vi "Robot参数整合一.vi"(7 "M4A数据":string[](array[string])=["", "", "", "", ""], 8 "A_Robot数据":string[](array[string])=["", "", "", "", "", "", "", "", "", "", "", "", "", "", ""], 10 "良率结算结果":string[](array[string]), 11 "Robot参数输入":string[](array[string])) -> (0 "Total数":string, 2 "数据整合输出":string[](array[string]), 3 "Robot数据输出结果":string[](array[string]))   [LabVIEW 2011]
panel:
  in  "数组":string[](array[string])=["Robot IP Set", "Robot Port Set", "PLC IP Set", "PLC Port Set", "Title Path", "Product", "StationID", "MachineSN", "HW", "GUI-Ver", "Robot-Ver", "Vision-Ver", "MachinMAC"]
  # "Product\n\nSN\n\nStationID\nMachineSN\nHW\nGUI-Ver\nRobot-Ver\nVision-Ver\n\nIP\n\nMachinMAC\n\nM4 Result\t\nblack wifi杓0.0\nM4 Fixture 1\n\nPoint,X,Y,Angle\nStartTime\nEndTime\nTime of CCD photographing\nM4 FPYR\nM4 Failing Rate\nM4 ReTest\nM4 CumRetestYield\nM4 ThroughtRate"
  # "Product\t\nStationID\t\nMachineSN\t\nHW\t\nGUI-Ver\t\nRobot-Ver\t\nVision-Ver\t\nIP\t\nMachinMAC\t\nPoint,X,Y,Angle\t\nStartTime\t\nEndTime\t\nTime of CCD photographing\t\nM4 FPYR\t\nM4 Failing Rate\t\nM4 ReTest\t\nM4 CumRetestYield\t\nM4 ThroughtRate\t\nRobot-OriginPosition\t\nRobot-CCD TopPosition\t\nRobot-CCD OriginPosition\t\nRobot-CCD ReTopPosition\t\nRobot-M4 TopPosition\t\nRobot-M4 OriginPosition\t\nRobot_M4 ReTopPosition\t\nRobot_CurrentPosition\t\nRobot-M4 TopPosition\t\nRobot-M4 OriginPosition\t\nRobot-M4 TopPosition\t\nM4_PassPosition\t\nM4_FailPosition"
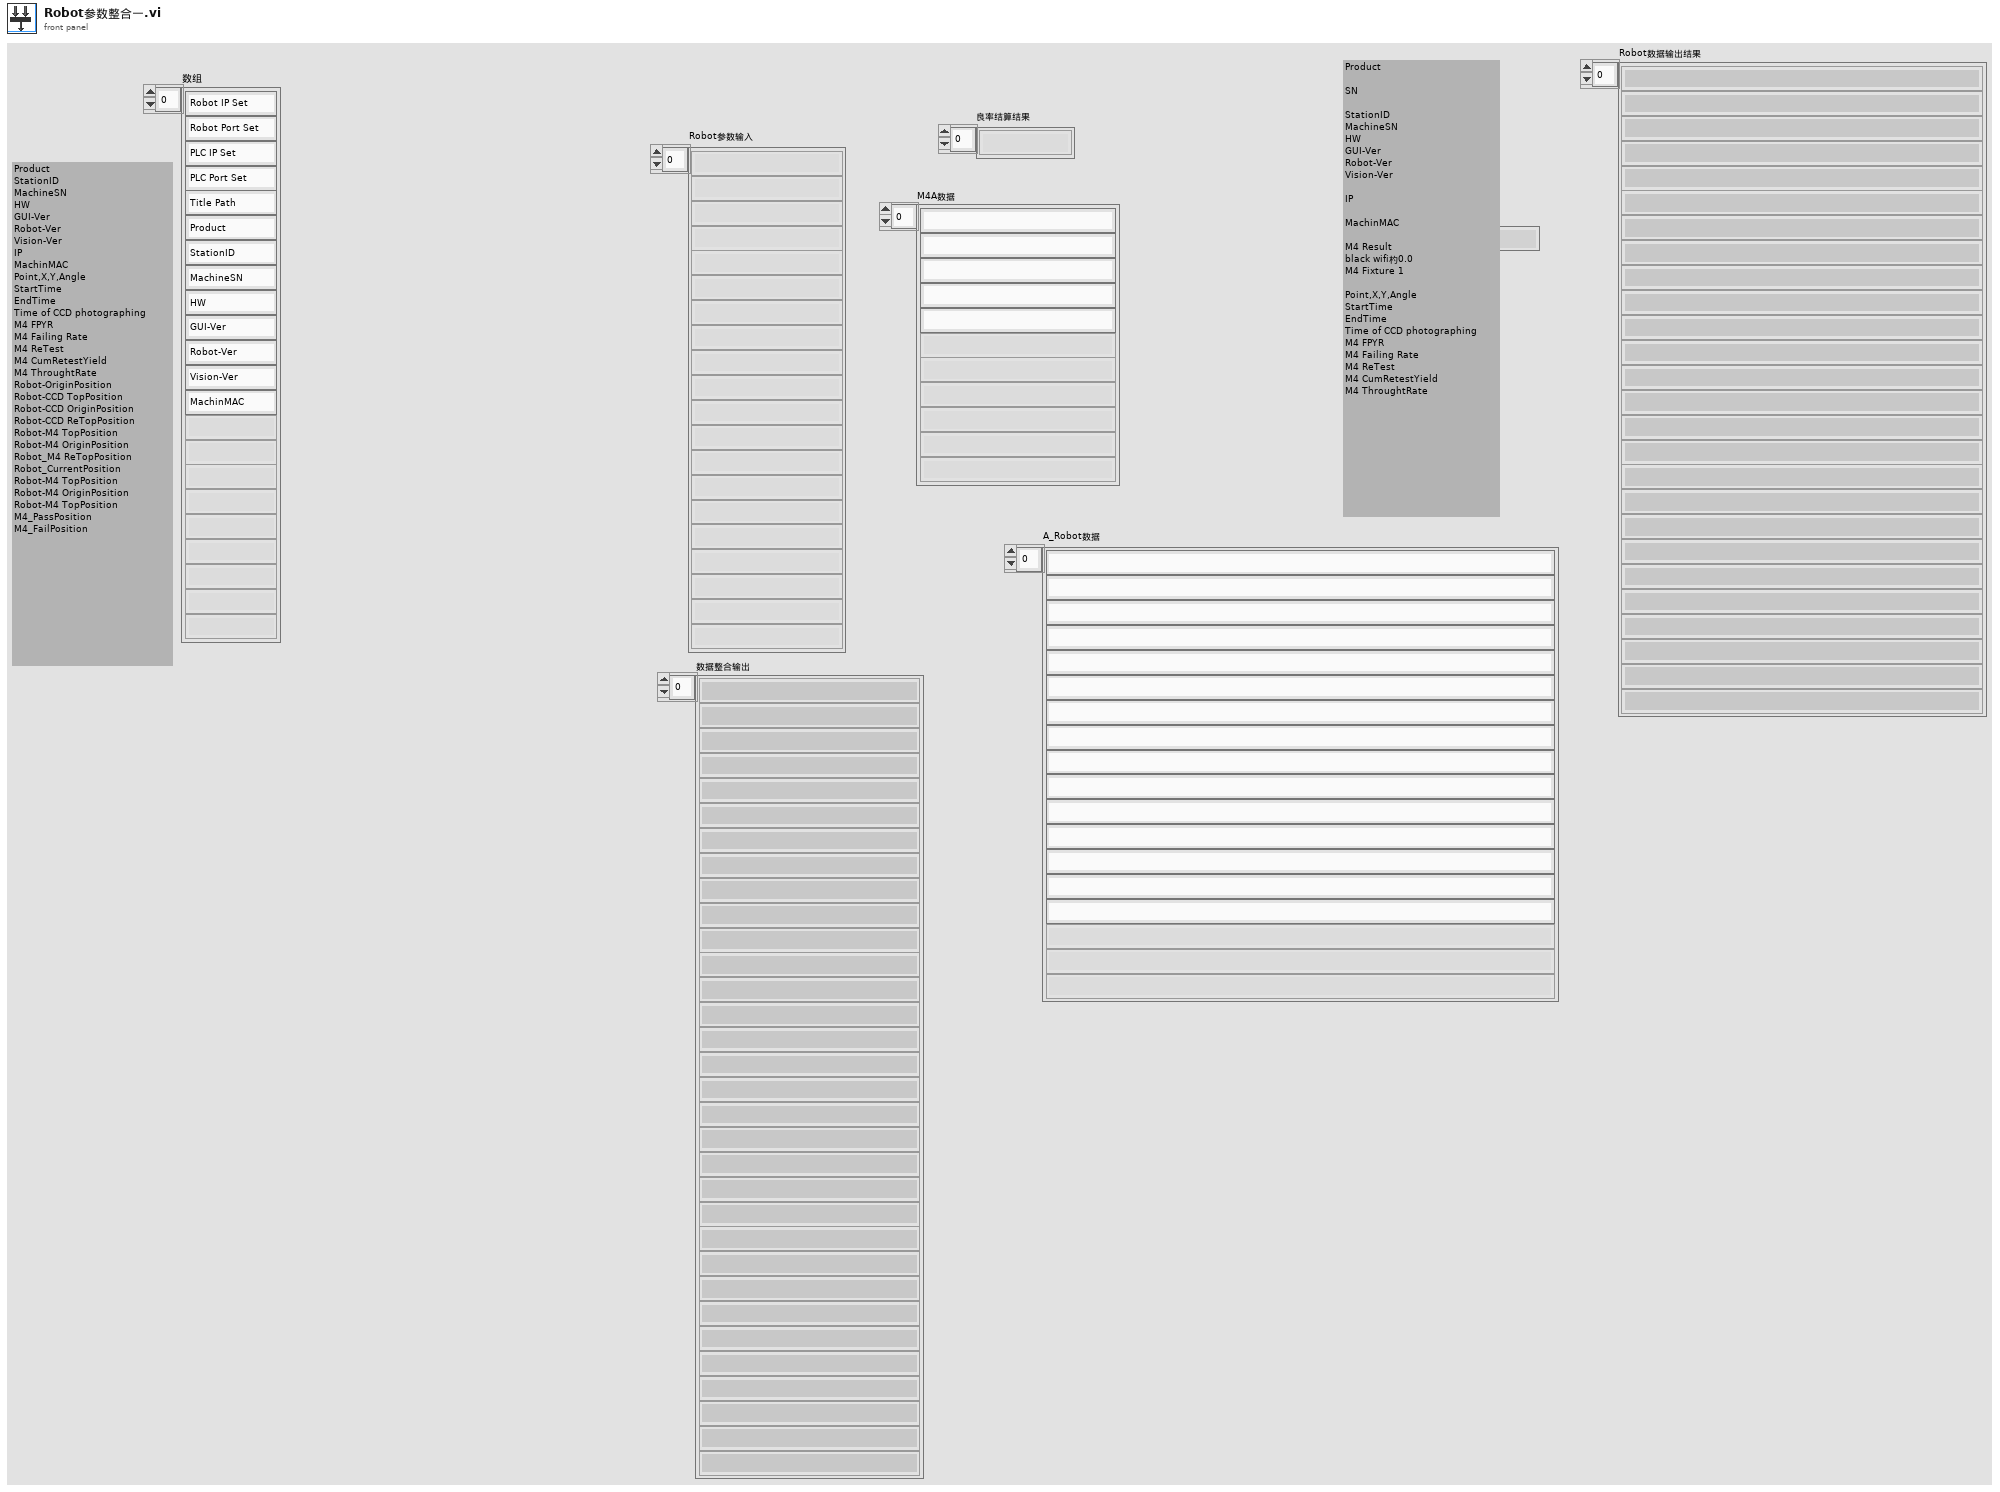
[diagram p1: front panel]
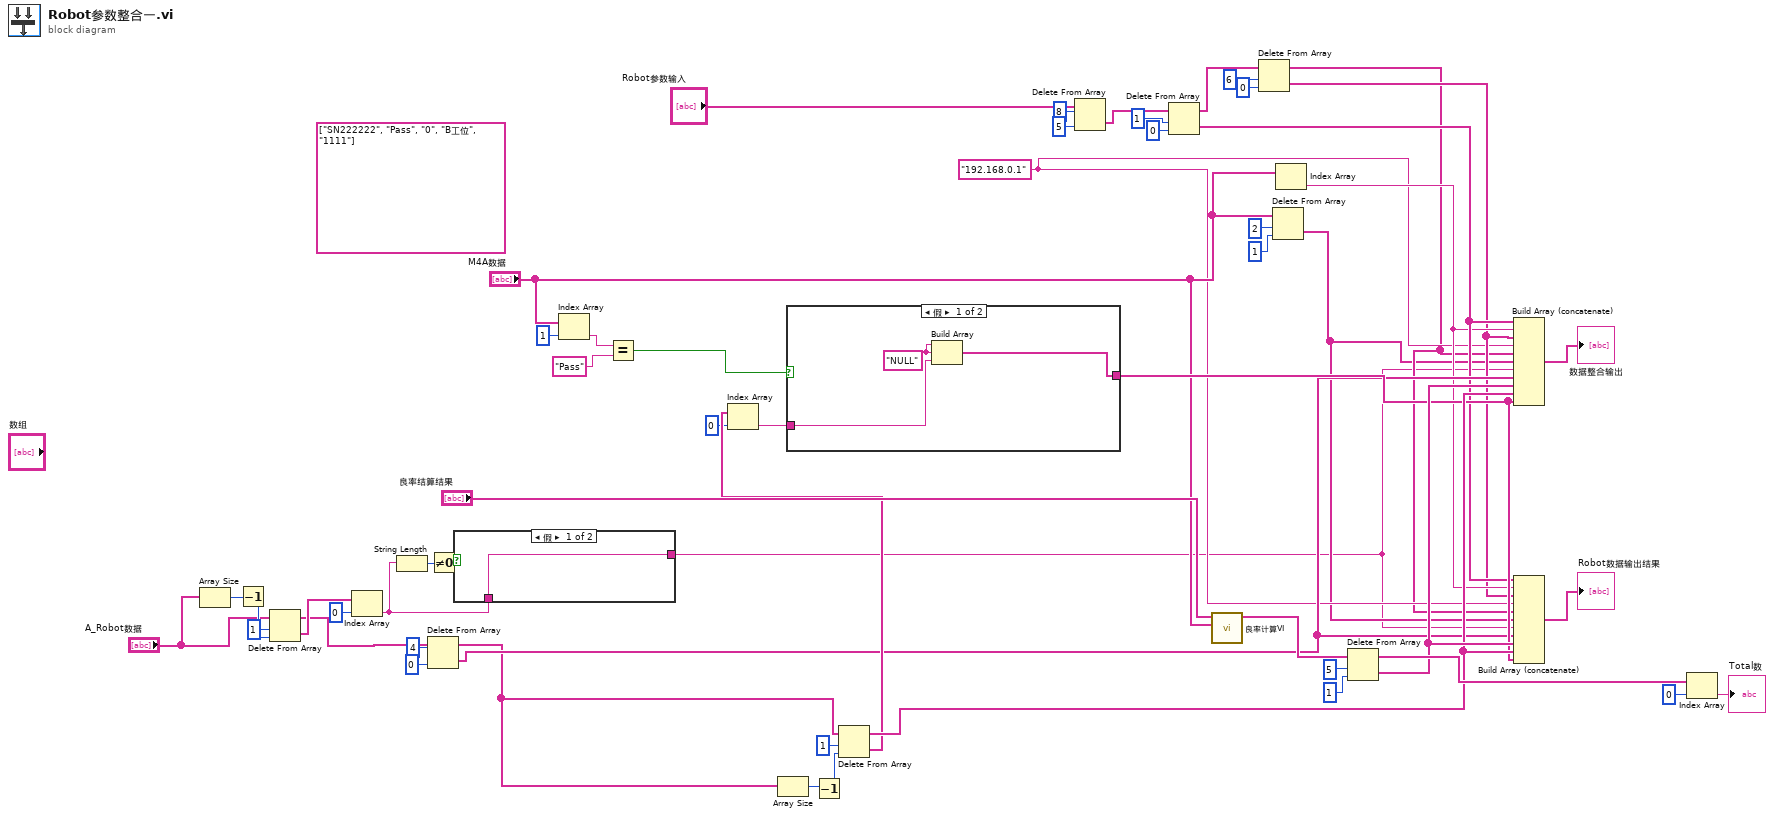
[diagram p0: block diagram]
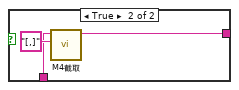
[diagram p2: hidden frame]
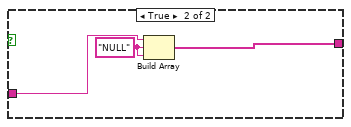
[diagram p3: hidden frame]
diagram:
  (unwired) string[] ["SN222222", "Pass", "0", "B工位", "1111"] ("M4A数据 2")
  w14 = "192.168.0.1"
  n1 = Array Size(array="A_Robot数据") -> (size(s)=w11:i32)
  n2 = Decrement(x=w11) -> (x-1=w10:i32)
  n3 = Delete From Array(array="A_Robot数据", length=1 ("长度"), index=w10) -> (deleted portion=w8:string[], array with subset deleted=w5:string[])
  n4 = Index Array(array=w8, index=0 ("索引")) -> (element=w3:string)
  n5 = String Length(string=w3) -> (length=w2:i32)
  n6 = Delete From Array(array=w5, length=4 ("长度"), index=0 ("索引")) -> (deleted portion=w29:string[], array with subset deleted=w28:string[])
  n7 = Not Equal To 0?(x=w2) -> (x != 0?=w1:bool)
  n8 = case shown="假" w1 {
    tunnel: [w56 w58] -> w4
    tunnel: w3 -> [w56 w57]
    frame False {
    }
    frame True {
      n9 = call "M4截取.vi"("匹配"="[,]", "字符輸入"=w57) -> ("输出"=w58:string)  [unwired: 9 in]
    }
  }
  n10 = Index Array(array="M4A数据", index=1 ("索引")) -> (element=w42:string)
  n11 = Equal?(x=w42, y="Pass") -> (x = y?=w36:bool)
  n12 = Array Size(array=w28) -> (size(s)=w40:i32)
  n13 = Decrement(x=w40) -> (x-1=w39:i32)
  n14 = Delete From Array(array=w28, length=1 ("长度"), index=w39) -> (deleted portion=w35:string[], array with subset deleted=w37:string[])
  n15 = Index Array(array=w35, index=0 ("索引")) -> (element=w33:string)
  n16 = case shown="假" w36 {
    tunnel: w33 -> [w62 w65]
    tunnel: [w61 w64] -> w32
    frame False {
      w60 = "NULL" ("元素")
      n17 = Build Array(w60, w60, w62) -> (w61:string[])
    }
    frame True {
      w63 = "NULL" ("元素")
      n18 = Build Array(w65, w63, w63) -> (w64:string[])
    }
  }
  n19 = Delete From Array(array="Robot参数输入", length=8 ("长度"), index=5 ("索引")) -> (deleted portion=w23:string[])  [unwired: 1 out]
  n20 = Delete From Array(array=w23, length=1 ("长度"), index=0 ("索引")) -> (deleted portion=w20:string[], array with subset deleted=w18:string[])
  n21 = call "良率计算VI.vi"("M4A数据"="M4A数据", "良率结算结果"="良率结算结果") -> ("判断结果输出"=w54:string[])  [unwired: 9 in]
  n22 = Delete From Array(array=w18, length=6 ("长度"), index=0 ("索引")) -> (deleted portion=w15:string[], array with subset deleted=w13:string[])
  n23 = Delete From Array(array="M4A数据", length=2 ("长度"), index=1 ("索引")) -> (deleted portion=w12:string[])  [unwired: 1 out]
  n24 = Index Array(array="M4A数据") -> (element=w19:string)  [unwired: 1 in]
  n25 = Delete From Array(array=w54, length=5 ("长度"), index=1 ("索引")) -> (deleted portion=w48:string[], array with subset deleted=w51:string[])
  n26 = Build Array (concatenate)(w20, w19, w15, w14, w13, w12, w4, w29, w48, w37, w32) -> (→"数据整合输出":string[])
  n27 = Build Array (concatenate)(w20, w19, w15, w14, w13, w12, w4, w29, w48, w37, w32) -> (→"Robot数据输出结果":string[])
  n28 = Index Array(array=w51, index=0 ("索引")) -> (element=→"Total数":string)
